vi "CAN Frame Array to Cluster.vi"(1 "CAN Frame Array In":u32[](array[numeric])=[0, 0, 0, 0, 0, 0]) -> (0 "CAN Frame Cluster Out":T1 {"Data" format="%.0x"; "DataLength" format="%.0x"; "InfoB" format="%.0x"; "InfoA" format="%.0x"; "Type" format="%.0x"; "Identifier" format="%.0x"; "Timestamp" format="%.0x"})   [LabVIEW 2016]
uses:
  Program Files (x86)/National Instruments/LabVIEW 2016/examples/robotics/EPOS2 CANOpen Driver/Low Level VIs/Typedefs/FPGA CAN Frame Cluster.ctl
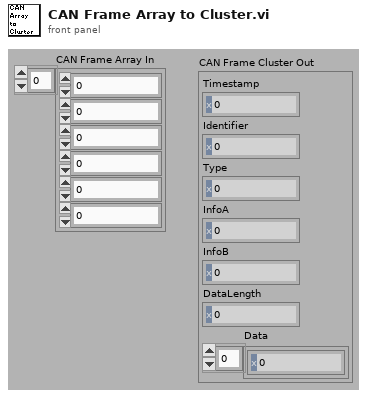
[diagram p1: front panel]
types:
  T1 = cluster{"Timestamp":u64, "Identifier":u32, "Type":u8, "InfoA":u8, "InfoB":u8, "DataLength":u8, "Data":u8[]}
  T2 = typedef "FPGA CAN Frame Cluster.ctl" = cluster{"Timestamp":u64, "Identifier":u32, "Type":u8, "InfoA":u8, "InfoB":u8, "DataLength":u8, "Data":u8[]}
  T3 = cluster{"CAN Frame Array In[0]":u32, "CAN Frame Array In[1]":u32, "CAN Frame Array In[2]":u32, "CAN Frame Array In[3]":u32, "CAN Frame Array In[4]":u32, "CAN Frame Array In[5]":u32}
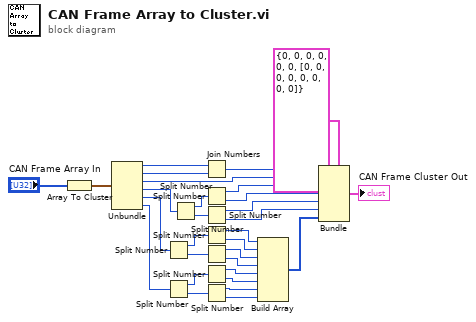
[diagram p0: block diagram]
diagram:
  n1 = Array To Cluster(array="CAN Frame Array In") -> (cluster=w8:T3)
  n2 = Unbundle(w8) -> ("CAN Frame Array In[0]"=w9:u32, "CAN Frame Array In[1]"=w10:u32, "CAN Frame Array In[2]"=w12:u32, "CAN Frame Array In[3]"=w13:u32, "CAN Frame Array In[4]"=w14:u32, "CAN Frame Array In[5]"=w21:u32)
  n3 = Split Number(x=w14) -> (hi(x)=w18:u16, lo(x)=w17:u16)
  n4 = Split Number(x=w21) -> (hi(x)=w19:u16, lo(x)=w20:u16)
  n5 = Split Number(x=w13) -> (hi(x)=w15:u16, lo(x)=w16:u16)
  n6 = Join Numbers(hi=w9, lo=w10) -> ((hi.lo)=w11:u64)
  n7 = Split Number(x=w15) -> (hi(x)=w4:u8, lo(x)=w3:u8)
  n8 = Split Number(x=w16) -> (hi(x)=w2:u8, lo(x)=w1:u8)
  n9 = Split Number(x=w18) -> (hi(x)=w22:u8, lo(x)=w23:u8)
  n10 = Split Number(x=w17) -> (hi(x)=w24:u8, lo(x)=w25:u8)
  n11 = Split Number(x=w19) -> (hi(x)=w26:u8, lo(x)=w27:u8)
  n12 = Split Number(x=w20) -> (hi(x)=w28:u8, lo(x)=w29:u8)
  n13 = Build Array(w22, w23, w24, w25, w26, w27, w28, w29) -> (w30:u8[])
  n14 = Bundle(cluster=T2 {"Timestamp"=0, "Identifier"=0, "Type"=0, "InfoA"=0, "InfoB"=0, "DataLength"=0, "Data"=[0, 0, 0, 0, 0, 0, 0, 0]} ("CAN Frame Cluster Out 2"), "Timestamp"=w11, "Identifier"=w12, "Type"=w4, "InfoA"=w3, "InfoB"=w2, "DataLength"=w1, "Data"=w30) -> (→"CAN Frame Cluster Out":T2)
